vi "GetTileCode.vi"() -> ()   [LabVIEW 2019, in "RT_Game.lvlib" / "Bouncer.lvclass"]
uses:
  Bouncer.lvclass
  Game/Game.lvclass
panel:
  out "TileCode 2":u16
  out "found?":bool
  out "TileNumber":u8
  out "error out":errorcluster
  in  "TileCode":string
  in  "error in (no error)":errorcluster
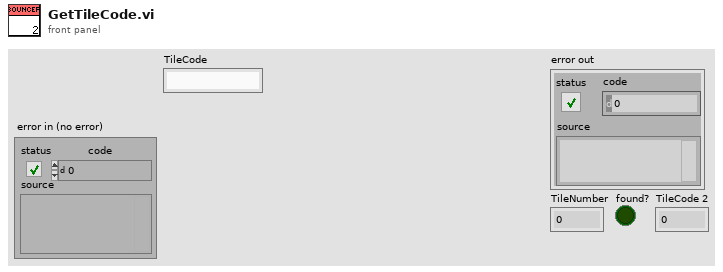
[diagram p1: front panel]
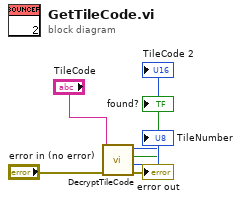
[diagram p0: block diagram]
diagram:
  n1 = call "DecryptTileCode.vi"("error in (no error)"="error in (no error)", "TileCode"="TileCode") -> ("error out"=→"error out":errorcluster, "TileNumber"=→"TileNumber":u8, "found?"=→"found?":bool, "TileCode"=→"TileCode 2":u16)  [unwired: 6 in]
